vi "预测成本.vi"() -> ()   [LabVIEW 2018]
uses:
  <vilib>/silver_ctls/ArrayMatrixCluster/Real Matrix NI_Silver.ctl
  <vilib>/Analysis/NI_AALPro.lvlib
panel:
  out "方程":string
  out "波形图":dbl[][](graph)
  out "系数":dbl[](array[numeric])
  out "均方根":dbl caption="残差"
  in  "Y":dbl[](array[numeric])=[150.0, 75.0, 120.0, 300.0, 50.0]
  out "H":T1
  in  "X2":dbl[](array[numeric])=[3.0, 3.2, 3.1, 2.8, 2.5]
  in  "X1":dbl[](array[numeric])=[295.0, 100.0, 200.0, 700.0, 60.0]
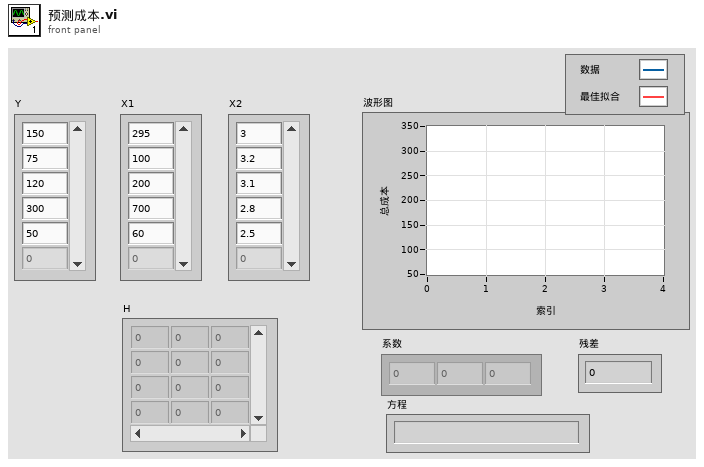
[diagram p1: front panel]
types:
  T1 = typedef "Real Matrix NI_Silver.ctl" = dbl[][]
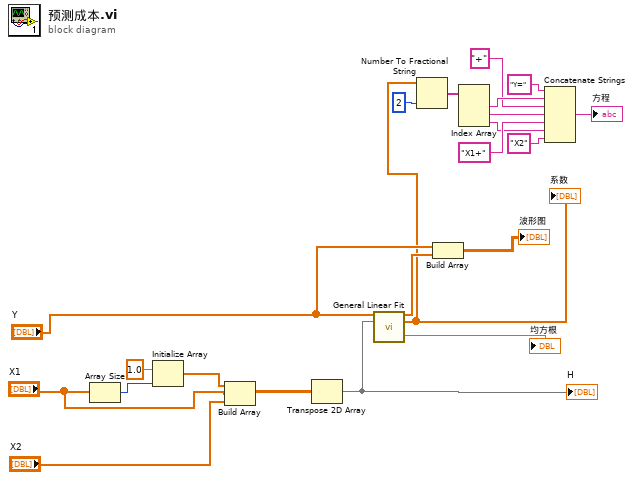
[diagram p0: block diagram]
diagram:
  n1 = Array Size(array="X1") -> (size(s)=w22:i32)
  n2 = Initialize Array(1.0 ("元素"), w22) -> (w20:dbl[])
  n3 = Build Array(w20, "X1", "X2") -> (w17:dbl[][])
  n4 = Transpose 2D Array(2D array=w17) -> (transposed array=w16:dbl[][])
  "H" <- w16
  n5 = call <vilib>:"General Linear Fit.vi"("Y"="Y", "H"=w16) -> ("Best Fit"=w14:dbl[], "Coefficients"=w10:dbl[], "residue"=→"均方根":dbl)  [unwired: 8 in, 3 out]
  "系数" <- w10
  n6 = Number To Fractional String(number=w10, precision (6)=i16 2 ("精度(6)")) -> (F-format string=w9:string[])  [unwired: 2 in]
  n7 = Build Array("Y", w14) -> (→"波形图":dbl[][])
  n8 = Index Array(array=w9) -> (element #1=w7:string, element #2=w5:string, element #3=w3:string)  [unwired: 3 in]
  n9 = Concatenate Strings("Y=" ("字符串"), w7, "+" ("字符串"), w5, "X1+" ("字符串"), w3, "X2" ("字符串")) -> (→"方程":string)
